vi "Write Selected DTRows.vi"(8 "error in (no error)":errorcluster, 10 "Selected DTRows":string[][](array[string]), 11 "Controller UI in":refnum<class "Controller UI.lvclass">) -> (0 "error out":errorcluster, 3 "Controller UI out":refnum<class "Controller UI.lvclass">)   [LabVIEW 2016, in "Controller UI.lvlib" / "Controller UI.lvclass"]
uses:
  <userlib>/Common Components/Controller UI/Controller UI.lvclass
  <userlib>/Common Components/Controller UI/Controller UI.lvclass/Controller UI.ctl
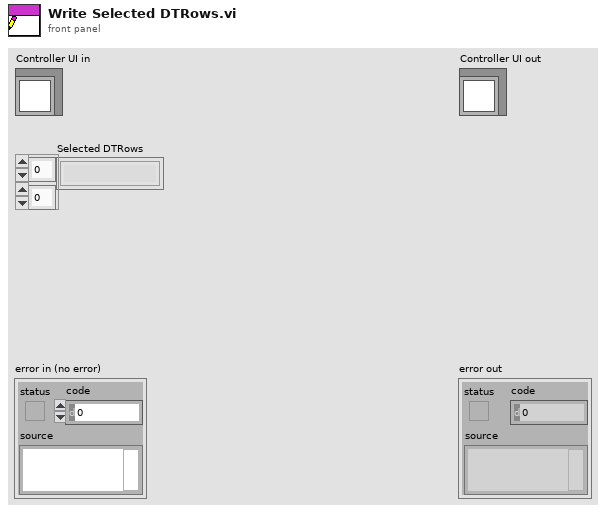
[diagram p1: front panel]
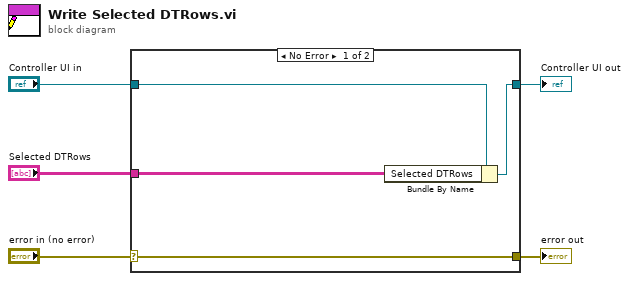
[diagram p0: block diagram]
diagram:
  n1 = case shown="No Error" "error in (no error)" {
    selector: "error in (no error)" -> [w9 w10]
    tunnel: [w9 w10] -> w4
    tunnel: [w7 w11] -> w2
    tunnel: "Controller UI in" -> [w8 w11]
    tunnel: "Selected DTRows" -> [w6 _]
    frame No Error {
      n2 = Bundle By Name(cluster=w8, "Selected DTRows"=w6) -> (w7:refnum<class "Controller UI.lvclass">)
    }
    frame Error {
    }
  }
  "error out" <- w4
  "Controller UI out" <- w2
